vi "draw_position_overlay.vi"(8 "error in (no error)":errorcluster, 10 "pixel positions":T1[](array[typedef]), 11 "Image in":refnum<class "Image.lvclass">) -> (0 "error out":errorcluster, 3 "Image out":refnum<class "Image.lvclass">)   [LabVIEW 2010, in "Image.lvclass"]
uses:
  Image.lvclass
  pixel_position_cluster.ctl
  ErrorController/ErrorController/class_data.vi
  ErrorController/ErrorController/ErrorController.lvclass
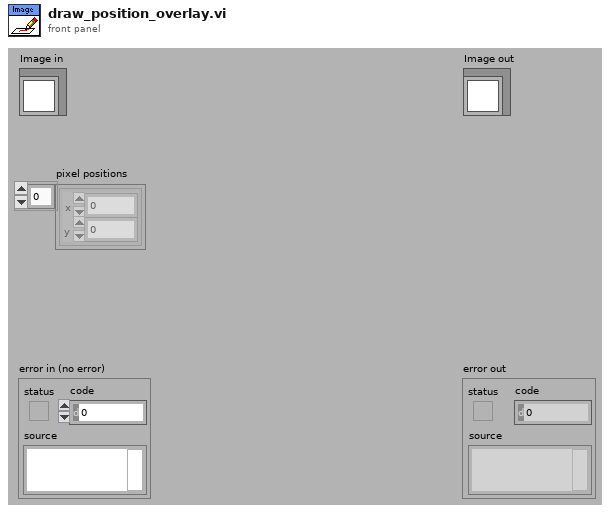
[diagram p1: front panel]
types:
  T1 = typedef "Image.lvclass/pixel_position_cluster.ctl" = cluster{"x":dbl, "y":dbl}
  T2 = typedef "IMAQ Image.ctl" = refnum<image>
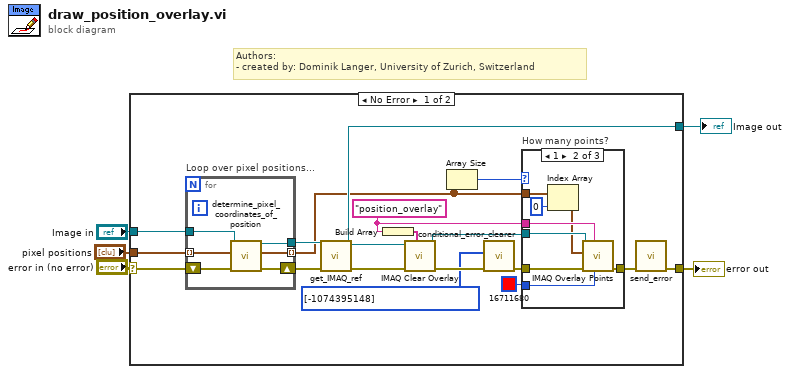
[diagram p0: block diagram]
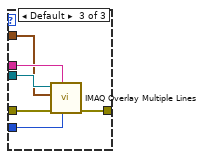
[diagram p3: hidden frame]
diagram:
  # "Authors: \n- created by: Dominik Langer, University of Zurich, Switzerland"
  n1 = case shown="No Error" "error in (no error)" {
    selector: "error in (no error)" -> [w24 w47]
    tunnel: [w7 w47] -> w4
    tunnel: [w17 w46] -> w2
    tunnel: "Image in" -> [w22 w46]
    tunnel: "pixel positions" -> [w23 _]
    frame No Error {
      w15 = "position_overlay"
      n2 = for "Loop over pixel positions..." {
        tunnel: w23 -> [w43] mode=indexing
        tunnel: w22 -> [w42]
        tunnel: [w41] -> w16
        shift-right: [w44] -> w20
        shift-left: w24 -> [w45]
        tunnel: [w40] -> w11 mode=indexing
        n3 = call "determine_pixel_coordinates_of_position.vi"("error in (no error)"=w45, "pixel position"=w43, "Image in"=w42) -> ("error out"=w44:errorcluster, "Point Coordinates"=w40:cluster{"X":dbl, "Y":dbl}, "Image out"=w41:refnum<class "Image.lvclass">)  [unwired: 6 in]
      }
      n4 = call-dynamic "get_IMAQ_ref.vi"("error in (no error)"=w20, "Image.lvclass in"=w16) -> ("error out"=w19:errorcluster, "Image"=w18:T2, "Image.lvclass out"=w17:refnum<class "Image.lvclass">)  [unwired: 5 in, 2 out]
      n5 = Build Array(w15) -> (w21:string[])
      n6 = call "IMAQ Clear Overlay"("Groups"=w21, "error in (no error)"=w19, "Image"=w18) -> ("error out"=w10:errorcluster, "Image Out"=w14:T2)  [unwired: 7 in]
      n7 = Array Size(array=w11) -> (size(s)=w12:i32)
      n8 = call "conditional_error_clearer.vi"("error in (no error)"=w10, "array of clearable error codes"=i32[] [-1074395148]) -> ("error out"=w9:errorcluster)  [unwired: 9 in]
      n9 = case "How many points?" shown="1" w12 {
        tunnel: w9 -> [w25 w33 w38]
        tunnel: w14 -> [_ w31 w37]
        tunnel: w15 -> [_ w30 w36]
        tunnel: w11 -> [_ w28 w35]
        tunnel: u32 16711680 ("Color") -> [_ w29 w34]
        tunnel: [w25 w32 w39] -> w6
        frame 0 {
        }
        frame 1 {
          n10 = Index Array(array=w28, index=0) -> (element=w26:cluster{"X":dbl, "Y":dbl})
          n11 = call "IMAQ Overlay Points"("Color"=w29, "Group"=w30, "error in (no error)"=w33, "Point"=w26, "Image"=w31) -> ("error out"=w32:errorcluster)  [unwired: 5 in, 1 out]
        }
        frame Default {
          n12 = call "IMAQ Overlay Multiple Lines"("Color"=w34, "Group"=w36, "error in (no error)"=w38, "Line End Points"=w35, "Image"=w37) -> ("error out"=w39:errorcluster)  [unwired: 5 in, 1 out]
        }
      }
      n13 = call "send_error.vi"("error in (no error)"=w6) -> ("error out"=w7:errorcluster)  [unwired: 10 in]
    }
    frame Error {
    }
  }
  "error out" <- w4
  "Image out" <- w2
